vi "_variant.vi"(6 "Add when NonExist?":bool, 8 "error in (no error)":errorcluster, 9 "default value (empty variant)":variant, 10 "name":string, 11 "DB Ref":T1) -> (0 "error out":errorcluster, 2 "value":variant, 3 "DB Ref (dup)":T1)   [LabVIEW 2014, in "TagDB(dev).lvlib"]
uses:
  TagDB(dev).lvlib
  tagDB_Def.ctl
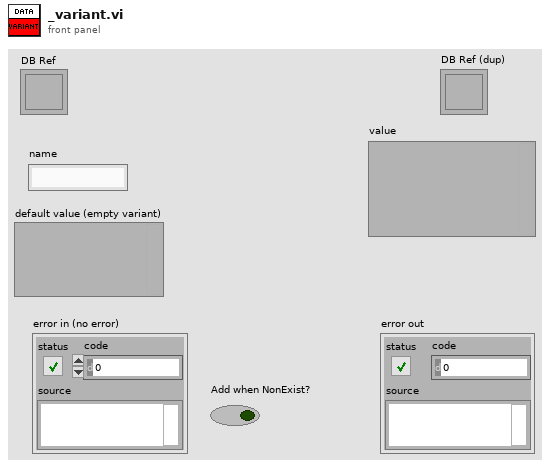
[diagram p1: front panel]
types:
  T1 = typedef "TagDB(dev).lvlib/tagDB_Def.ctl" = refnum<k1>
  T2 = typedef "TagDB(dev).lvlib/_DEF-DATA.ctl" = cluster{"data hashmap":variant, "DataChangeFlag":i64, "ItemChangeFlag":i64, "name":string, "Tag Adding Lock?":bool}
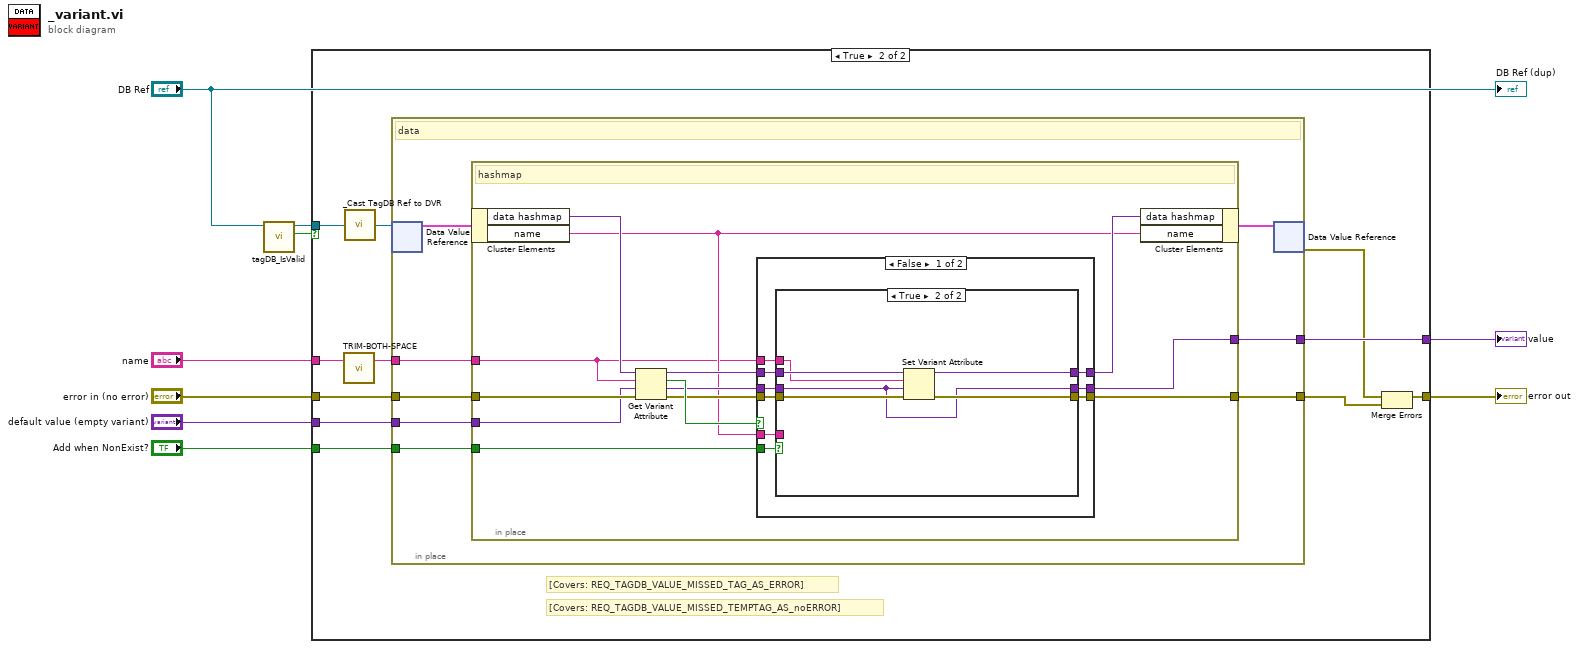
[diagram p0: block diagram]
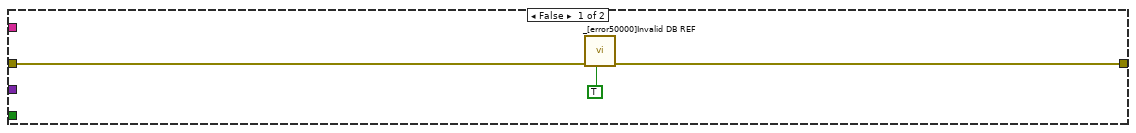
[diagram p2: hidden frame]
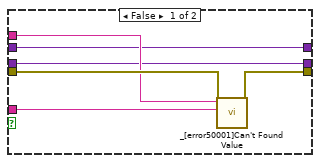
[diagram p3: hidden frame]
diagram:
  n1 = call "tagDB_IsValid.vi"("DB Ref in"="DB Ref") -> ("valid?"=w1:bool, "DB Ref out"=w2:T1)  [unwired: 8 in, 1 out]
  n2 = case shown="True" w1 {
    tunnel: "error in (no error)" -> [w12 w23]
    tunnel: "name" -> [_ w14]
    tunnel: [w11 w22] -> w6
    tunnel: "Add when NonExist?" -> [_ w19]
    tunnel: "default value (empty variant)" -> [_ w18]
    tunnel: [_ w17] -> w3
    tunnel: w2 -> [_ w16]
    frame False {
      n3 = call "_[error50000]Invalid DB REF.vi"("Force Gen?"=TRUE, "error in (no error)"=w12) -> ("error out"=w11:errorcluster)  [unwired: 9 in]
    }
    frame True {
      # "[Covers: REQ_TAGDB_VALUE_MISSED_TEMPTAG_AS_noERROR]"
      # "[Covers: REQ_TAGDB_VALUE_MISSED_TAG_AS_ERROR]"
      n4 = call "TRIM-BOTH-SPACE.vi"("name in"=w14) -> ("name out"=w13:string)  [unwired: 2 in]
      n5 = call "_Cast TagDB Ref to DVR.vi"("TagDB"=w16) -> ("DVR"=w21:refnum<data-value>)  [unwired: 4 in]
      n6 = in-place {
        in-place-border: w23 -> [w30]
        in-place-border: [w29] -> w20
        in-place-border: w13 -> [w27]
        in-place-border: w19 -> [w26]
        in-place-border: w18 -> [w25]
        in-place-border: [w24] -> w17
        # "data"
        n7 = in-place-dvr #1(w21) -> (w28:T2)  [unwired: 1 out]
        n8 = in-place {
          in-place-border: w30 -> [w44]
          in-place-border: [w40] -> w29
          in-place-border: w27 -> [w32]
          in-place-border: w26 -> [w36]
          in-place-border: w25 -> [w37]
          in-place-border: [w35] -> w24
          # "hashmap"
          n9 = in-place-cluster #2(w28) -> ("data hashmap"=w43:variant, "name"=w33:string)
          n10 = Get Variant Attribute(Variant=w43, name=w32, default value (empty Variant)=w37, error in=w44) -> (duplicate Variant=w39:variant, found=w42:bool, value=w34:variant, error out=w41:errorcluster)
          n11 = case shown="False" w42 {
            tunnel: w41 -> [w53 w68]
            tunnel: [w52 w68] -> w40
            tunnel: w32 -> [w51 _]
            tunnel: w39 -> [w48 w67]
            tunnel: [w49 w67] -> w38
            tunnel: w36 -> [w50 _]
            tunnel: [w47 w66] -> w35
            tunnel: w34 -> [w46 w66]
            tunnel: w33 -> [w45 _]
            frame False {
              n12 = case shown="True" w50 {
                tunnel: w53 -> [w59 w62]
                tunnel: [w58 w63] -> w52
                tunnel: w51 -> [w57 w60]
                tunnel: [w56 w64] -> w49
                tunnel: w48 -> [w56 w65]
                tunnel: [w55 w61] -> w47
                tunnel: w46 -> [w55 w61]
                tunnel: w45 -> [w54 _]
                frame False {
                  n13 = call "_[error50001]Can't Found Value.vi"("error in (no error)"=w59, "db name"=w54, "value name"=w57) -> ("error out"=w58:errorcluster)  [unwired: 8 in]
                }
                frame True {
                  n14 = Set Variant Attribute(Variant=w65, name=w60, value=w61, error in=w62) -> (Variant out=w64:variant, error out=w63:errorcluster)  [unwired: 1 out]
                }
              }
            }
            frame True {
            }
          }
          n15 = in-place-cluster #2("data hashmap"=w38, "name"=w33) -> (w31:T2)
        }
        n16 = in-place-dvr #1(w31) -> (w15:errorcluster)  [unwired: 1 out]
      }
      n17 = Merge Errors(w15, w20) -> (w22:errorcluster)
    }
  }
  "error out" <- w6
  "value" <- w3
  "DB Ref (dup)" <- "DB Ref"
